vi "Open References to Shared Variables.vi"(8 "error in (no error)":errorcluster, 10 "Process Data":T2={"Write URLs"={"URLs"=[]}, "Read URLs"={"URLs"=[]}, "Write SV FIFO"="", "Read SV FIFO"="", "Status SV FIFO"="", "Status Notifier"="", "Update Rate"=10}, 11 "SV Data":T1={"Status notifier"=refnum, "Write FIFO ref"=refnum, "Read FIFO ref"=refnum, "Status FIFO ref"=refnum, "Update Rate"=1, "Write Refs by Type"={"DBL Write"=[]}, "Read Refs by Type"={"DBL Read"=[]}, "WriteSize"=0, "ReadSize"=0}) -> (0 "error out":errorcluster, 3 "SV Data":T1={"Status notifier"=refnum, "Write FIFO ref"=refnum, "Read FIFO ref"=refnum, "Status FIFO ref"=refnum, "Update Rate"=1, "Write Refs by Type"={"DBL Write"=[]}, "Read Refs by Type"={"DBL Read"=[]}, "WriteSize"=0, "ReadSize"=0})   [LabVIEW 2020, in "Shared Variable Interface.lvlib"]
uses:
  Shared Variable Interface.lvlib
  Shared DataTypes/SV Process Data.ctl
  Shared DataTypes/URLs.ctl
  SV Process Configuration.ctl
  DataTypes/DBL.lvlib
panel:
  # "Out"
  # "In"
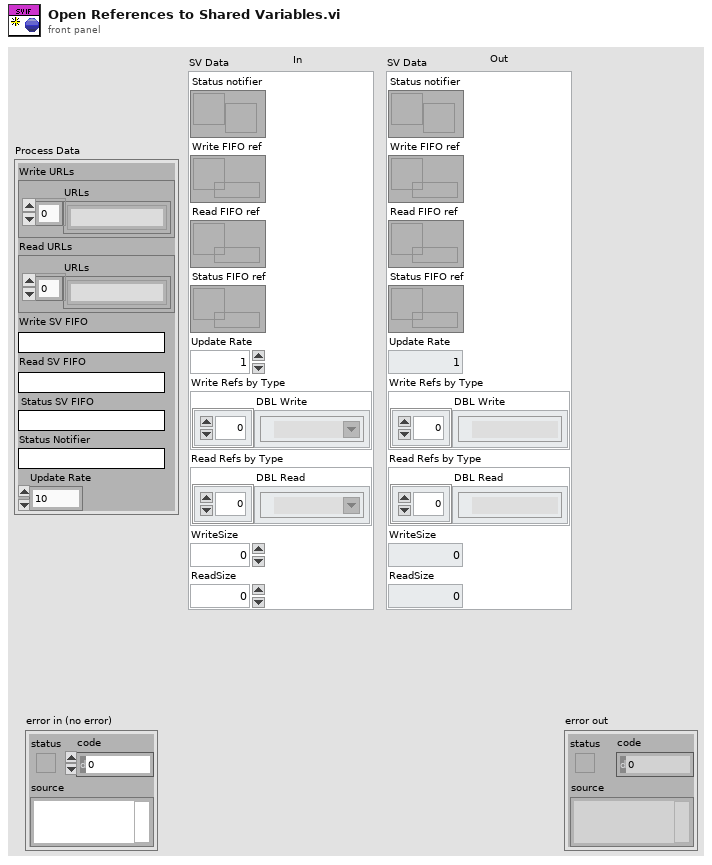
[diagram p1: front panel]
types:
  T1 = typedef "Shared Variable Interface.lvlib/SV Process Configuration.ctl" = cluster{"Status notifier":refnum<notifier>, "Write FIFO ref":refnum<k33>, "Read FIFO ref":refnum<k33>, "Status FIFO ref":refnum<k33>, "Update Rate":u32, "Write Refs by Type":cluster{"DBL Write":refnum<k21>[]}, "Read Refs by Type":cluster{"DBL Read":refnum<k21>[]}, "WriteSize":i32, "ReadSize":i32}
  T2 = typedef "SV Process Data.ctl" = cluster{"Write URLs":T3, "Read URLs":T3, "Write SV FIFO":string, "Read SV FIFO":string, "Status SV FIFO":string, "Status Notifier":string, "Update Rate":u32}
  T3 = typedef "URLs.ctl" = cluster{"URLs":string[]}
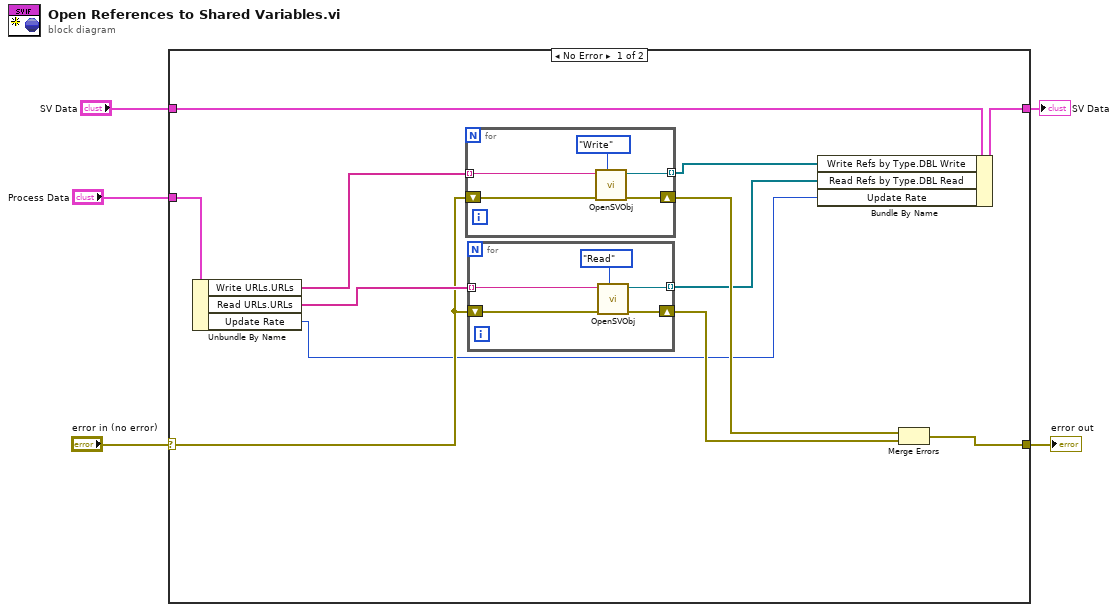
[diagram p0: block diagram]
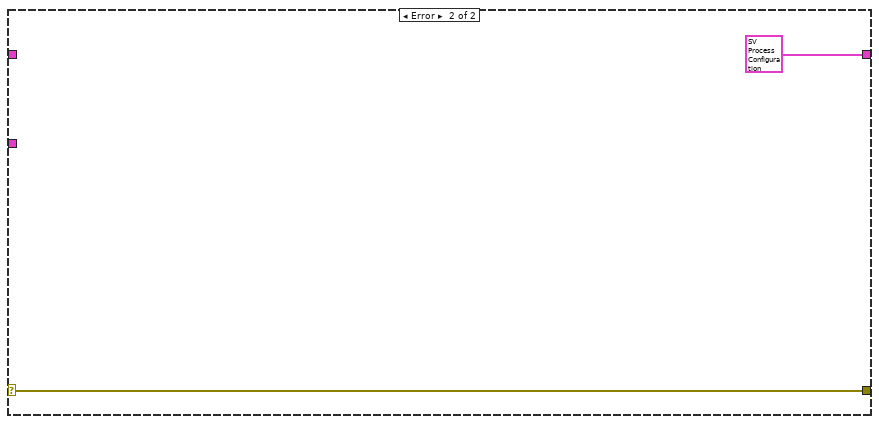
[diagram p2: hidden frame]
diagram:
  n1 = case shown="No Error" "error in (no error)" {
    selector: "error in (no error)" -> [w7 w29]
    tunnel: [w17 w29] -> w4
    tunnel: [w15 T1 {"Status notifier"=refnum, "Write FIFO ref"=refnum, "Read FIFO ref"=refnum, "Status FIFO ref"=refnum, "Update Rate"=1, "Write Refs by Type"={"DBL Write"=[]}, "Read Refs by Type"={"DBL Read"=[]}, "WriteSize"=0, "ReadSize"=0} ("SV Data")] -> w1
    tunnel: "Process Data" -> [w16 _]
    tunnel: "SV Data" -> [w8 _]
    frame No Error {
      n2 = Unbundle By Name(w16) -> ("Write URLs.URLs"=w14:string[], "Read URLs.URLs"=w11:string[], "Update Rate"=w6:u32)
      n3 = for {
        tunnel: w14 -> [w23] mode=indexing
        tunnel: [w27] -> w10 mode=indexing
        shift-right: [w26] -> w13
        shift-left: w7 -> [w25]
        n4 = call "OpenSVObj.vi"("AccessType"=enum16{"Read", "Write"}."Write", "error in"=w25, "SVref"=w23) -> ("error out"=w26:errorcluster, "SVref"=w27:refnum<k21>)  [unwired: 7 in]
      }
      n5 = for {
        tunnel: w11 -> [w18] mode=indexing
        tunnel: [w22] -> w9 mode=indexing
        shift-right: [w21] -> w12
        shift-left: w7 -> [w20]
        n6 = call "OpenSVObj.vi"("AccessType"=enum16{"Read", "Write"}."Read", "error in"=w20, "SVref"=w18) -> ("error out"=w21:errorcluster, "SVref"=w22:refnum<k21>)  [unwired: 7 in]
      }
      n7 = Bundle By Name(cluster=w8, "Write Refs by Type.DBL Write"=w10, "Read Refs by Type.DBL Read"=w9, "Update Rate"=w6) -> (w15:T1)
      n8 = Merge Errors(w13, w12) -> (w17:errorcluster)
    }
    frame Error {
    }
  }
  "error out" <- w4
  "SV Data" <- w1
